vi "Release Messaging Structure.vi"(8 "error in (no error)":errorcluster) -> (0 "error out":errorcluster)   [LabVIEW 2010, in "Launcher.lvlib"]
uses:
  Launcher.lvlib
  Error Handler/Error Handler.lvlib
  Error Handler/Event Ref FGV Command Enum.ctl
  Shutdown Event FGV Command.ctl
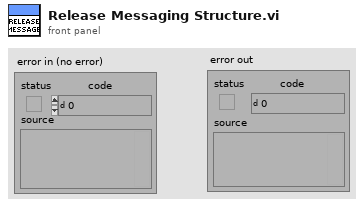
[diagram p1: front panel]
types:
  T1 = typedef "Launcher.lvlib/Shutdown Event FGV Command.ctl" = enum16{"Create Event", "Get Event Ref", "Release Event"}
  T2 = typedef "Error Handler.lvlib/Event Ref FGV Command Enum.ctl" = enum16{"Create Event", "Get Event Ref", "Release Event"}
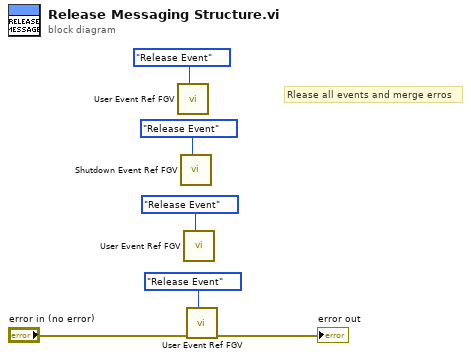
[diagram p0: block diagram]
diagram:
  # "Rlease all events and merge erros"
  n1 = call "User Event Ref FGV.vi"("Command"=Event_Ref_FGV_Command_Enum."Release Event") -> ()  [unwired: 9 in, 2 out]
  n2 = call "Shutdown Event Ref FGV.vi"("Command"=Shutdown_Event_FGV_Command."Release Event") -> ()  [unwired: 9 in, 2 out]
  n3 = call "User Event Ref FGV.vi"("Command"=Event_Ref_FGV_Command_Enum."Release Event") -> ()  [unwired: 9 in, 2 out]
  n4 = call "User Event Ref FGV.vi"("Command"=Event_Ref_FGV_Command_Enum."Release Event", "error in (no error)"="error in (no error)") -> ("error out"=→"error out":errorcluster)  [unwired: 8 in, 1 out]
